vi "parse_FP_mode.vi"(1 "line index":i32) -> (0 "output string":string)   [LabVIEW 2016]
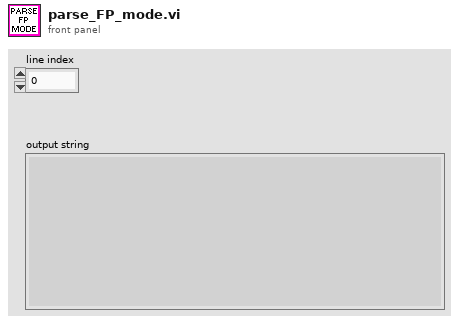
[diagram p1: front panel]
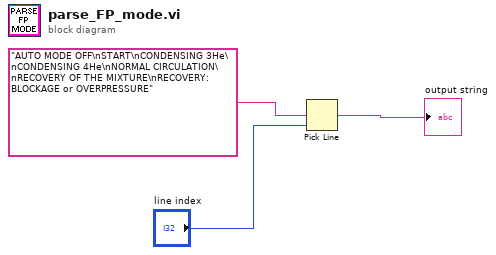
[diagram p0: block diagram]
diagram:
  n1 = Pick Line(multi-line string="AUTO MODE OFF\nSTART\nCONDENSING 3He\nCONDENSING 4He\nNORMAL CIRCULATION\nRECOVERY OF THE MIXTURE\nRECOVERY: BLOCKAGE or OVERPRESSURE", line index="line index") -> (output string=→"output string":string)  [unwired: 1 in]
